vi "Read HaltRole 4.vi"(8 "error in (no error)":errorcluster, 11 "HaltPlay in":refnum<class "HaltPlay.lvclass">) -> (0 "error out":errorcluster, 2 "HaltRole":refnum<class "HaltRole.lvclass">, 3 "HaltPlay out":refnum<class "HaltPlay.lvclass">)   [LabVIEW 2023, in "HaltPlay.lvclass"]
uses:
  HaltPlay.lvclass
  HaltRole_class/HaltRole.lvclass
  HaltPlay.lvclass/HaltPlay.ctl
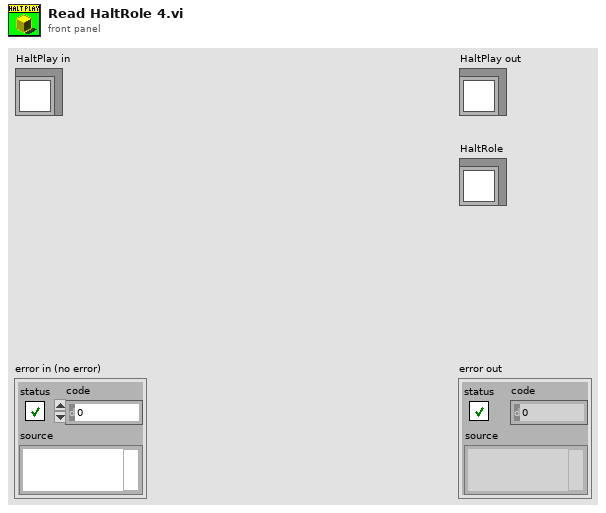
[diagram p1: front panel]
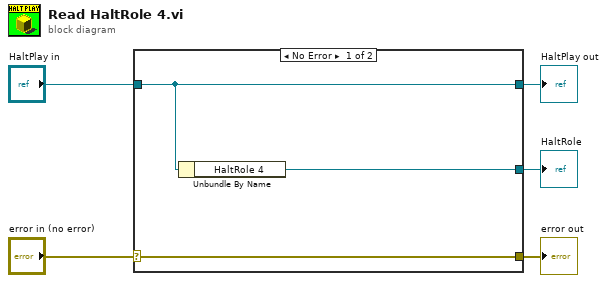
[diagram p0: block diagram]
diagram:
  n1 = case shown="No Error" "error in (no error)" {
    selector: "error in (no error)" -> [w8 w9]
    tunnel: [w8 w9] -> w4
    tunnel: [w7 w10] -> w2
    tunnel: "HaltPlay in" -> [w7 w10]
    tunnel: [w6 _] -> w1
    frame No Error {
      n2 = Unbundle By Name(w7) -> ("HaltRole 4"=w6:refnum<class "HaltRole.lvclass">)
    }
    frame Error {
    }
  }
  "error out" <- w4
  "HaltPlay out" <- w2
  "HaltRole" <- w1
